vi "Control de Movimiento y Vibracion_f.vi"(3 "Error In":errorcluster, 4 "SetFrec.":dbl) -> (0 "Error Out":errorcluster, 1 "Muy cerca":bool, 2 "Frecuencia":dbl format="%#_5g", 5 "A":dbl, 6 "FFT":cluster{"f0":dbl, "df":dbl, "magnitude":dbl[]}[](graph) caption="fft")   [LabVIEW 2018]
uses:
  <vilib>/measure/matone.llb/Extract Single Tone Information N Chan.vi
  <vilib>/measure/maspectr.llb/FFT Power Spectrum and PSD for N Chan.vi
  <vilib>/measure/NI_MAPro.lvlib
panel:
  out "Filtered Signal":dynamicdata(graph)
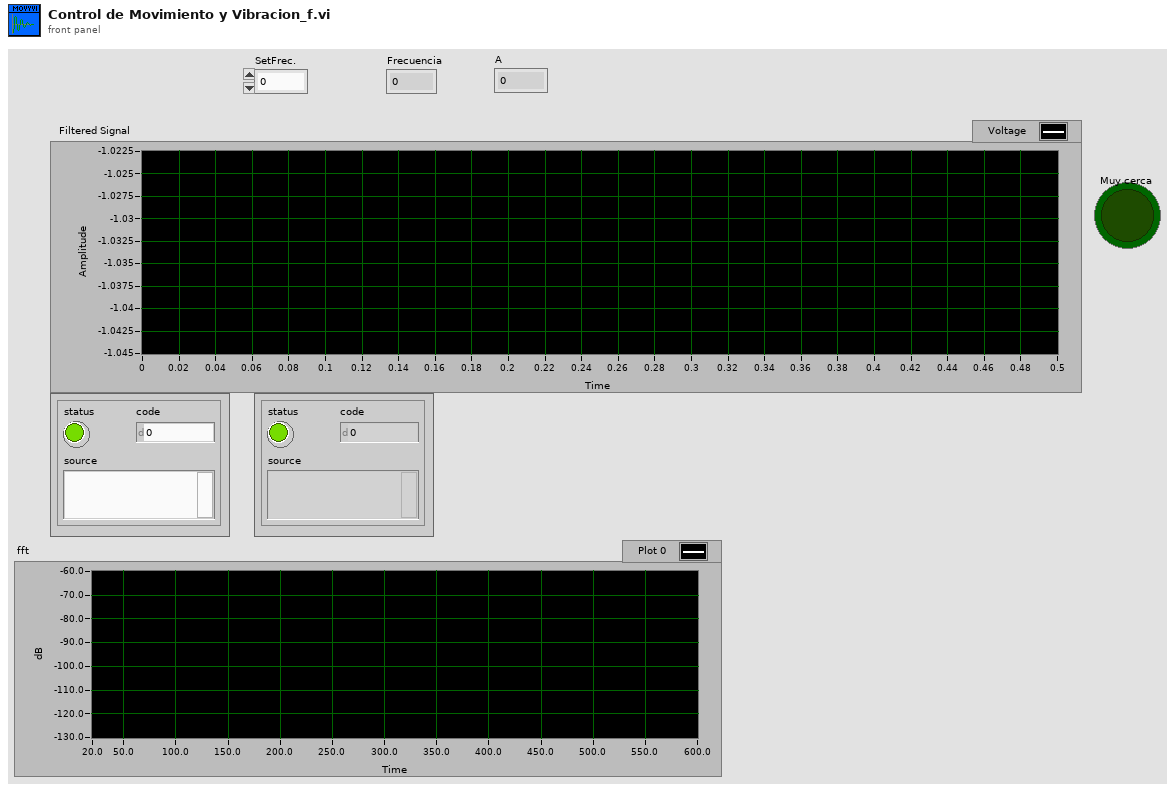
[diagram p1: front panel]
types:
  T1 = cluster{"averaging mode":enum16{"No averaging", "Vector averaging", "RMS averaging", "Peak hold"}, "weighting mode":enum16{"Linear", "Exponential"}, "number of averages":u32}
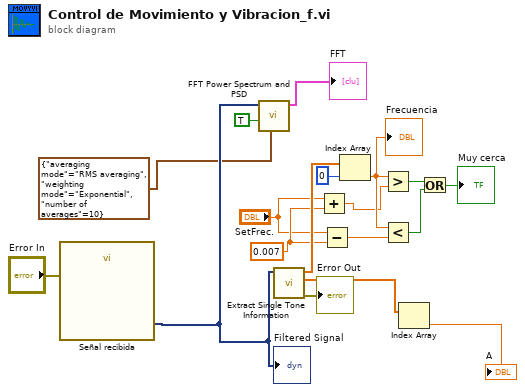
[diagram p0: block diagram]
diagram:
  w2 = 0.007
  n1 = call "Señal recibida"("error in"="Error In") -> ("data"=w9:dynamicdata)  [unwired: 15 in, 3 out]
  "Filtered Signal" <- w9
  n2 = call-poly <vilib>:"FFT Power Spectrum and PSD.vi"("averaging parameters"=T1 {"averaging mode"=enum."RMS averaging", "weighting mode"=enum."Exponential", "number of averages"=10}, "dB On (F)"=TRUE, "time signals"=w9) -> ("Power Spectrum / PSD"=→"FFT":cluster{"f0":dbl, "df":dbl, "magnitude":dbl[]}[])  [unwired: 5 in, 3 out]
  n3 = call-poly <vilib>:"Extract Single Tone Information.vi"("time signals in"=w9) -> ("error out"=→"Error Out":errorcluster, "detected amplitudes"=w5:dbl[], "detected frequencies"=w18:dbl[])  [unwired: 5 in, 3 out]
  n4 = Add(x="SetFrec.", y=w2) -> (x+y=w4:dbl)
  n5 = Subtract(x="SetFrec.", y=w2) -> (x-y=w3:dbl)
  n6 = Index Array(array=w18, index=0) -> (element=w16:dbl)
  "Frecuencia" <- w16
  n7 = Greater?(x=w16, y=w4) -> (0:w15:bool)
  n8 = Less?(x=w16, y=w3) -> (x < y?=w14:bool)
  n9 = Index Array(array=w5) -> (element=→"A":dbl)  [unwired: 1 in]
  n10 = Or(x=w15, y=w14) -> (x .or. y?=→"Muy cerca":bool)
